vi "Altura_Sol.vi"(0 "Grados":i32, 1 "Declinación":dbl, 2 "Minutos":i32, 3 "Segundos":i32, 4 "Ángulo Horario":dbl) -> (5 "Altura del Sol":dbl)   [LabVIEW 2020]
panel:
  # "Latitud"
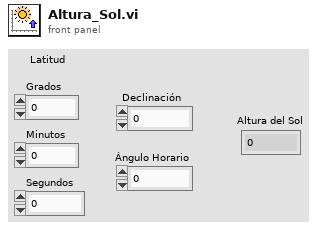
[diagram p1: front panel]
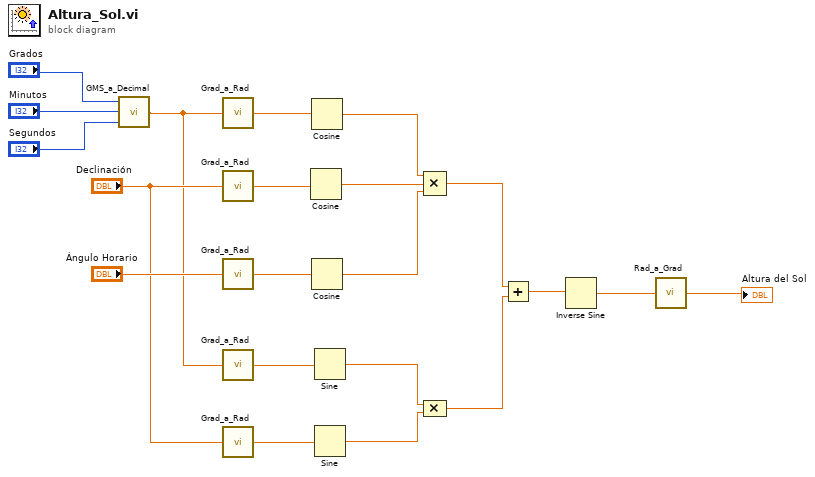
[diagram p0: block diagram]
diagram:
  n1 = call "GMS_a_Decimal.vi"("Segundos"="Segundos", "Minutos"="Minutos", "Grados"="Grados") -> ("Decimal"=w6:dbl)
  n2 = call "Grad_a_Rad.vi"("Grados"=w6) -> ("Radianes"=w21:dbl)
  n3 = call "Grad_a_Rad.vi"("Grados"="Declinación") -> ("Radianes"=w20:dbl)
  n4 = call "Grad_a_Rad.vi"("Grados"="Ángulo Horario") -> ("Radianes"=w19:dbl)
  n5 = call "Grad_a_Rad.vi"("Grados"=w6) -> ("Radianes"=w17:dbl)
  n6 = call "Grad_a_Rad.vi"("Grados"="Declinación") -> ("Radianes"=w16:dbl)
  n7 = Cosine(x=w20) -> (cos(x)=w13:dbl)
  n8 = Cosine(x=w21) -> (cos(x)=w14:dbl)
  n9 = Cosine(x=w19) -> (cos(x)=w12:dbl)
  n10 = Sine(x=w17) -> (sin(x)=w11:dbl)
  n11 = Sine(x=w16) -> (sin(x)=w10:dbl)
  n12 = Compound Arithmetic op=MULTIPLY(w14, w13, w12) -> (w9:dbl)
  n13 = Compound Arithmetic op=MULTIPLY(w11, w10) -> (w8:dbl)
  n14 = Add(x=w9, y=w8) -> (x+y=w7:dbl)
  n15 = Inverse Sine(1:w7) -> (0:w2:dbl)
  n16 = call "Rad_a_Grad.vi"("Radianes"=w2) -> ("Grados"=→"Altura del Sol":dbl)
